vi "Find Edge.vi"(0 "FSM in":refnum<class "FSM.Graph.lvclass">, 5 "From":string, 7 "To":string, 9 "Type":string, 11 "error in (no error)":errorcluster) -> (4 "FSM thru":refnum<class "FSM.Graph.lvclass">, 6 "Edge Index":i32, 15 "error out":errorcluster)   [LabVIEW 2015, in "FSM.Graph.lvclass"]
uses:
  FSM.Graph.lvclass
  FSM.Graph.lvclass/FSM.Graph.ctl
  FSM.Edge/FSM.Edge.lvclass/FSM.Edge.ctl
  FSM.Label/FSM.Label.lvclass/FSM.Label.ctl
  FSM.Edge/Read SourceName.vi
  FSM.Edge/Read TargetName.vi
  FSM.Edge/Read Type.vi
  FSM.Edge/Read Label.vi
  FSM.Label/Read Text.vi
  FSM.Label/FSM.Label.lvclass
  FSM.Edge/FSM.Edge.lvclass
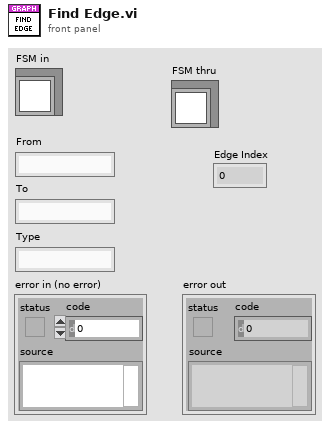
[diagram p1: front panel]
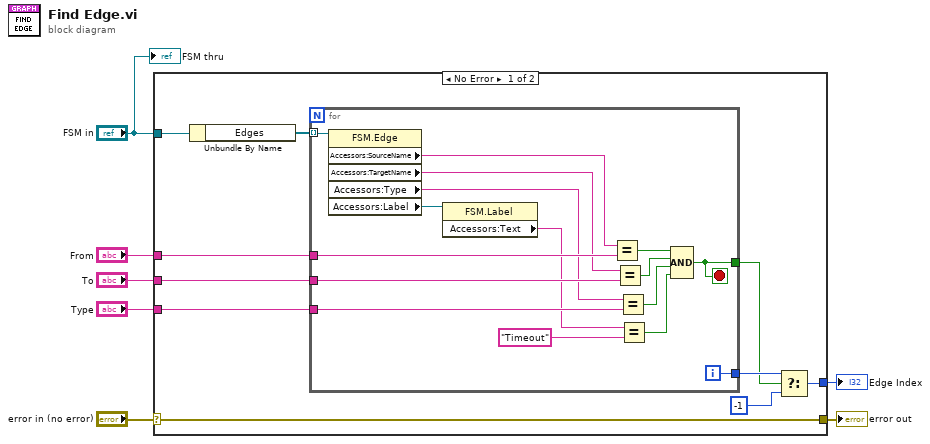
[diagram p0: block diagram]
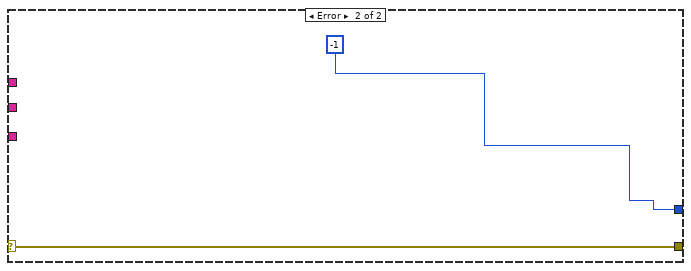
[diagram p2: hidden frame]
diagram:
  n1 = case shown="No Error" "error in (no error)" {
    selector: "error in (no error)" -> [w17 w35]
    tunnel: [w17 w35] -> w6
    tunnel: "FSM in" -> [w13 _]
    tunnel: [w16 -1] -> w4
    tunnel: "From" -> [w11 _]
    tunnel: "To" -> [w10 _]
    tunnel: "Type" -> [w9 _]
    frame No Error {
      n2 = Unbundle By Name(w13) -> ("Edges"=w12:refnum<class "FSM.Edge.lvclass">[])
      n3 = for {
        tunnel: w12 -> [w32] mode=indexing
        tunnel: [w33] -> w15
        tunnel: w11 -> [w31]
        tunnel: w10 -> [w28]
        tunnel: w9 -> [w26]
        tunnel: [w22] -> w8
        i -> [w33]
        stop <- w22 stop-if-true
        n4 = property class="FSM.Edge"(reference=w32) -> ("Accessors:SourceName"=w30:string, "Accessors:TargetName"=w29:string, "Accessors:Type"=w27:string, "Accessors:Label"=w21:refnum<class "FSM.Label.lvclass">)  [unwired: 1 in, 2 out]
        n5 = property class="FSM.Label"(reference=w21) -> ("Accessors:Text"=w20:string)  [unwired: 1 in, 2 out]
        n6 = Equal?(x=w30, y=w31) -> (x = y?=w25:bool)
        n7 = Equal?(x=w29, y=w28) -> (x = y?=w24:bool)
        n8 = Equal?(x=w27, y=w26) -> (x = y?=w23:bool)
        n9 = Equal?(x=w20, y="Timeout") -> (x = y?=w18:bool)
        n10 = Compound Arithmetic op=AND(w25, w24, w23, w18) -> (w22:bool)
      }
      n11 = Select(t=w15, s=w8, f=-1) -> (s? t:f=w16:i32)
    }
    frame Error {
    }
  }
  "error out" <- w6
  "Edge Index" <- w4
  "FSM thru" <- "FSM in"
